vi "Read Hardware Handles.vi"(8 "error in":errorcluster, 11 "Execution Unit in":refnum<class "Execution Unit.lvclass">) -> (0 "error out":errorcluster, 2 "hardware handles":T1, 3 "Execution Unit out":refnum<class "Execution Unit.lvclass">)   [LabVIEW 2023, in "Ballard MIL-STD-1553 Engine Support.lvlib" / "Implementation.lvlib" / "Execution Unit.lvclass"]
uses:
  Execution Unit.lvclass
  Custom Device/Hardware Handles.ctl
  Execution Unit.lvclass/Execution Unit.ctl
  Custom Device/Custom Device.lvlib
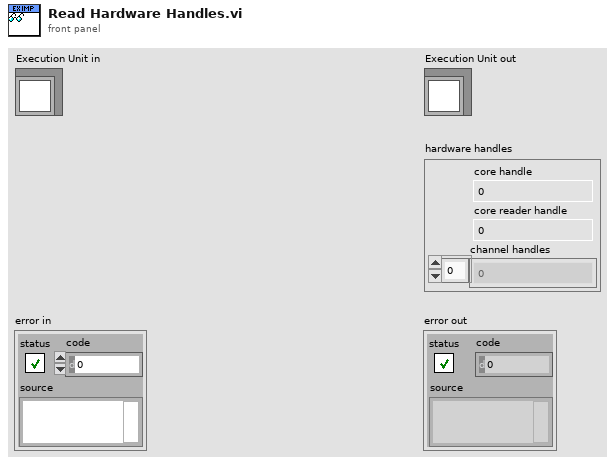
[diagram p1: front panel]
types:
  T1 = typedef "Ballard MIL-STD-1553 Engine Support.lvlib/Custom Device.lvlib/Hardware Handles.ctl" = cluster{"core handle":u64, "core reader handle":u64, "channel handles":u64[]}
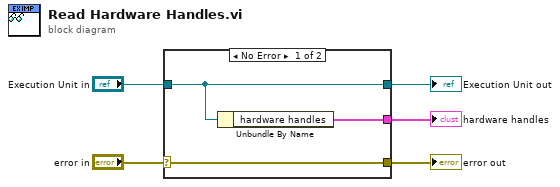
[diagram p0: block diagram]
diagram:
  n1 = case shown="No Error" "error in" {
    selector: "error in" -> [w8 w9]
    tunnel: [w8 w9] -> w4
    tunnel: [w7 w10] -> w2
    tunnel: "Execution Unit in" -> [w7 w10]
    tunnel: [w6 _] -> w1
    frame No Error {
      n2 = Unbundle By Name(w7) -> ("hardware handles"=w6:T1)
    }
    frame Error {
    }
  }
  "error out" <- w4
  "Execution Unit out" <- w2
  "hardware handles" <- w1
